vi "Is Array Element.vi"(8 "error in (no error)":errorcluster, 11 "Config Element in":refnum<class "Config Element.lvclass">) -> (0 "error out":errorcluster, 2 "Array Element":bool, 3 "Config Element out":refnum<class "Config Element.lvclass">)   [LabVIEW 2020, in "CDM-Config.lvlib" / "Config Element.lvclass"]
uses:
  Config Element.lvclass
  Config Element.lvclass/Config Element.ctl
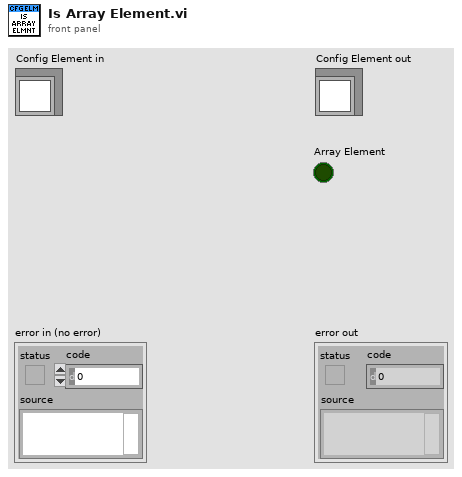
[diagram p1: front panel]
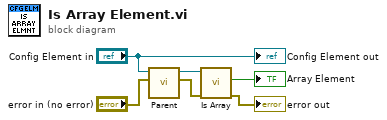
[diagram p0: block diagram]
diagram:
  n1 = call "Parent.vi"("error in (no error)"="error in (no error)", "Config Element in"="Config Element in") -> ("error out"=w4:errorcluster, "Parent"=w5:refnum<class "Config Element.lvclass">)  [unwired: 8 in]
  n2 = call "Is Array.vi"("error in (no error)"=w4, "Config Element in"=w5) -> ("error out"=→"error out":errorcluster, "Array"=→"Array Element":bool)  [unwired: 7 in, 1 out]
  "Config Element out" <- "Config Element in"
